vi "Serialize - JSON.vi"(8 "error in (no error)":errorcluster, 11 "CRDS Data in":refnum<class "CRDS Data.lvclass">) -> (0 "error out":errorcluster, 2 "Serialized JSON":string, 3 "CRDS Data out":refnum<class "CRDS Data.lvclass">)   [LabVIEW 2014, in "CRDS Lib.lvlib" / "CRDS Data.lvclass"]
uses:
  CRDS Data.lvclass
  CRDS Data.lvclass/CRDS Data.ctl
  Cell/CRDS Cell Data.lvclass
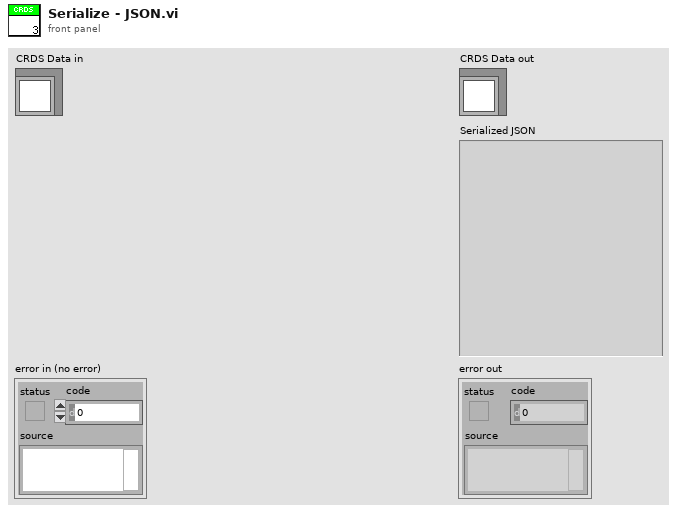
[diagram p1: front panel]
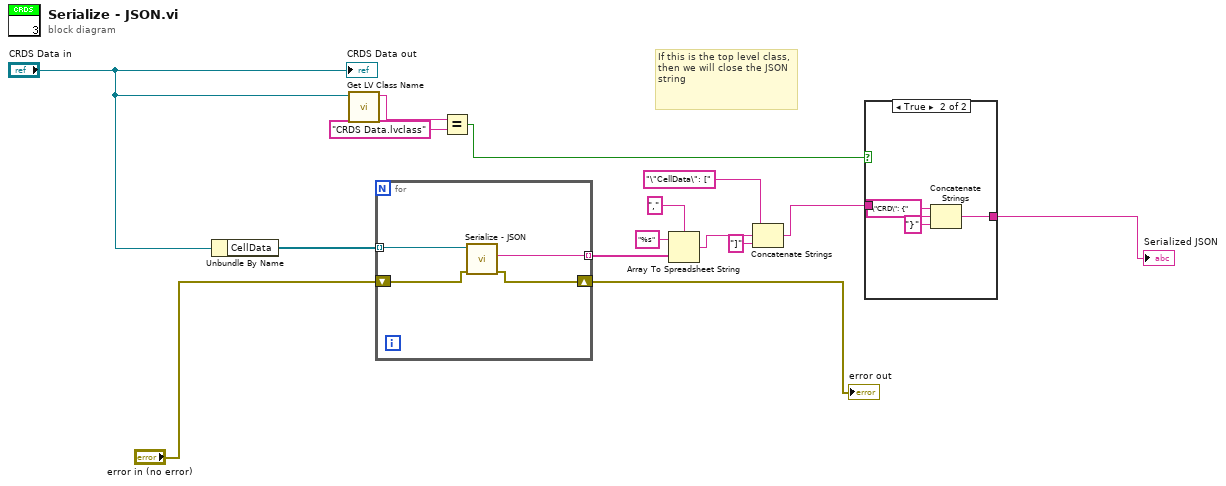
[diagram p0: block diagram]
diagram:
  # "If this is the top level class, then we will close the JSON string"
  n1 = Unbundle By Name("CRDS Data in") -> ("CellData"=w15:refnum<class "CRDS Cell Data.lvclass">[])
  n2 = call <vilib>:"Get LV Class Name.vi"("object"="CRDS Data in") -> ("class name"=w8:string)  [unwired: 9 in, 1 out]
  n3 = for {
    tunnel: w15 -> [w19] mode=indexing
    tunnel: [w18] -> w14 mode=indexing
    shift-right: [w16] -> w2
    shift-left: "error in (no error)" -> [w17]
    n4 = call-dynamic "Serialize - JSON.vi"("error in"=w17, "CRDS Cell Data in"=w19) -> ("error out"=w16:errorcluster, "Serialized JSON"=w18:string)  [unwired: 7 in, 1 out]
  }
  "error out" <- w2
  n5 = Equal?(x=w8, y="CRDS Data.lvclass") -> (x = y?=w3:bool)
  n6 = Array To Spreadsheet String(delimiter (Tab)=",", array=w14, 3:"%s" ("format string")) -> (spreadsheet string=w11:string)
  n7 = Concatenate Strings("\"CellData\": [" ("string"), w11, "]" ("string")) -> (w6:string)
  n8 = case shown="True" w3 {
    tunnel: w6 -> [w20 w24]
    tunnel: [w20 w21] -> w4
    frame False {
    }
    frame True {
      n9 = Concatenate Strings("\"CRD\": {" ("string"), w24, "}" ("string")) -> (w21:string)
    }
  }
  "Serialized JSON" <- w4
  "CRDS Data out" <- "CRDS Data in"
